vi "select.vi"() -> ()   [LabVIEW 2017]
panel:
  in  "?":bool
  out "Температура":dbl
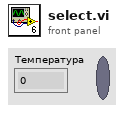
[diagram p1: front panel]
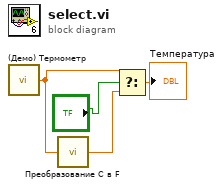
[diagram p0: block diagram]
diagram:
  n1 = call "(Демо) Термометр.vi"() -> ("Температура"=w3:dbl)  [unwired: 1 in]
  n2 = call "Преобразование C в F.vi"("Град C"=w3) -> ("Град F"=w2:dbl)
  n3 = Select(t=w3, s="?", f=w2) -> (s? t:f=→"Температура":dbl)
